vi "newTestStandVariable.vi"(0 "Engine Reference":refnum<k7>, 5 "Sequence File Ref":refnum<k7>, 7 "Variable Type":i32(ring)=1 items=["PropValType_Container", "PropValType_String", "PropValType_Boolean", "PropValType_Number", "PropValType_NamedType", "PropValType_Reference", "PropValType_Array"], 9 "Variable Name":string="Locals.Logs", 11 "error in":errorcluster, 12 "Variable Value":variant, 13 "Array?":bool, 14 "Empty array?":bool) -> (4 "Engine Reference(out)":refnum<k7>, 6 "Sequence File Ref(out)":refnum<k7>, 15 "error out":errorcluster)   [LabVIEW 2010]
doc: "This VI is used to create a TestStand variable. The variable type needs to be specified by selecting the type in the Variable Type enum control."
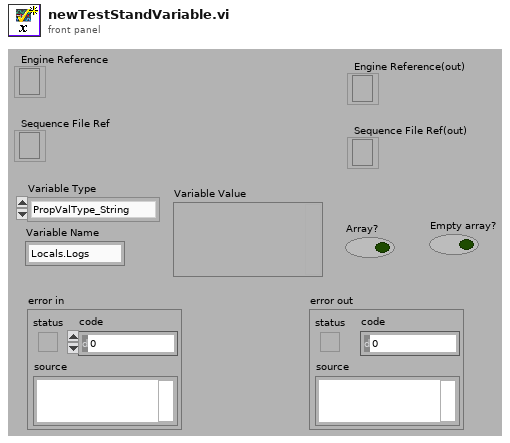
[diagram p1: front panel]
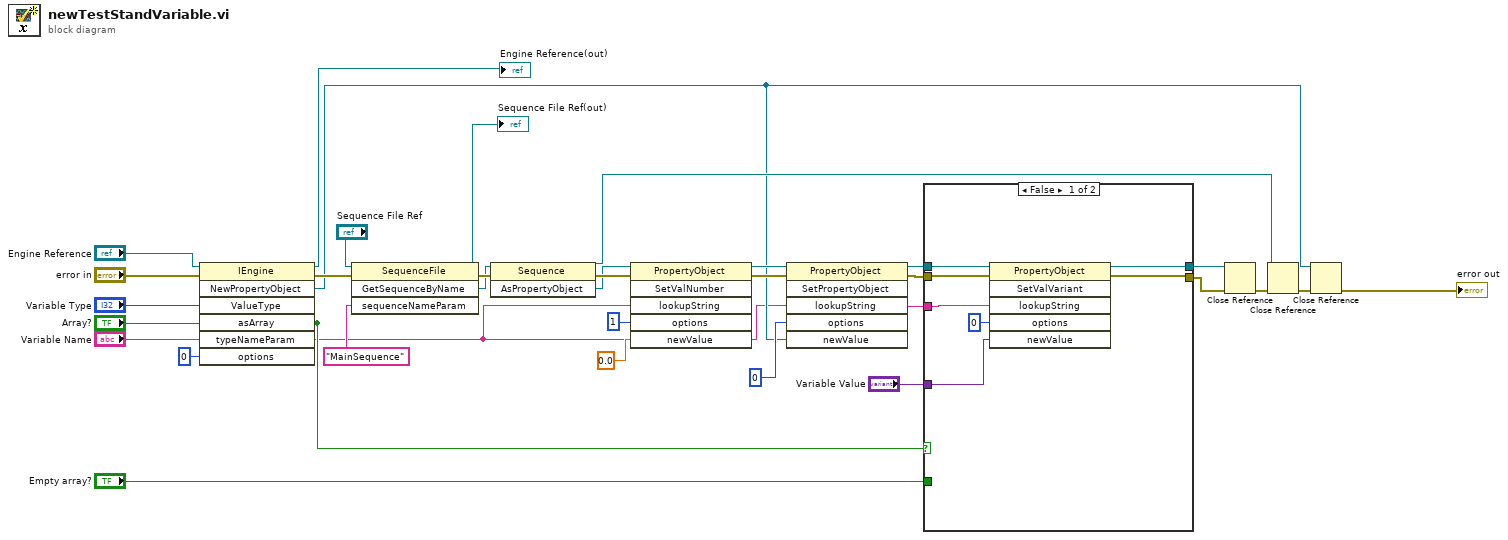
[diagram p0: block diagram]
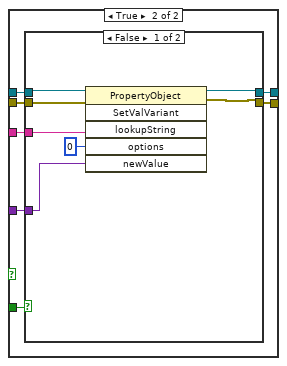
[diagram p2: hidden frame]
diagram:
  n1 = invoke class="IEngine" method="NewPropertyObject"(reference="Engine Reference", error in="error in", "ValueType"="Variable Type", "asArray"="Array?", "typeNameParam"="Variable Name", "options"=0) -> (reference out=→"Engine Reference(out)":refnum<k7>, error out=w11:errorcluster, "NewPropertyObject"=w10:refnum<k7>)  [unwired: 1 in, 4 out]
  n2 = invoke class="SequenceFile" method="GetSequenceByName"(reference="Sequence File Ref", error in=w11, "sequenceNameParam"="MainSequence") -> (reference out=→"Sequence File Ref(out)":refnum<k7>, error out=w17:errorcluster, "GetSequenceByName"=w15:refnum<k7>)  [unwired: 1 in, 1 out]
  n3 = invoke class="Sequence" method="AsPropertyObject"(reference=w15, error in=w17) -> (reference out=w19:refnum<k7>, error out=w13:errorcluster, "AsPropertyObject"=w12:refnum<k7>)  [unwired: 1 in]
  n4 = invoke class="PropertyObject" method="SetValNumber"(reference=w12, error in=w13, "lookupString"="Variable Name", "options"=1, "newValue"=0.0) -> (reference out=w23:refnum<k7>, error out=w21:errorcluster)  [unwired: 1 in, 4 out]
  n5 = invoke class="PropertyObject" method="SetPropertyObject"(reference=w23, error in=w21, "lookupString"="Variable Name", "options"=0, "newValue"=w10) -> (reference out=w8:refnum<k7>, error out=w5:errorcluster)  [unwired: 1 in, 4 out]
  n6 = case shown="False" "Array?" {
    tunnel: w8 -> [w38 w45]
    tunnel: [w37 w44] -> w7
    tunnel: "Empty array?" -> [_ w41]
    tunnel: [w36 w42] -> w4
    tunnel: w5 -> [w35 w43]
    tunnel: "Variable Name" -> [w33 w40]
    tunnel: "Variable Value" -> [w34 w39]
    frame False {
      n7 = invoke class="PropertyObject" method="SetValVariant"(reference=w38, error in=w35, "lookupString"=w33, "options"=0, "newValue"=w34) -> (reference out=w37:refnum<k7>, error out=w36:errorcluster)  [unwired: 1 in, 4 out]
    }
    frame True {
      n8 = case shown="False" w41 {
        tunnel: w45 -> [w52 w54]
        tunnel: [w49 w54] -> w44
        tunnel: w43 -> [w51 w53]
        tunnel: [w48 w53] -> w42
        tunnel: w40 -> [w50 _]
        tunnel: w39 -> [w46 _]
        frame False {
          n9 = invoke class="PropertyObject" method="SetValVariant"(reference=w52, error in=w51, "lookupString"=w50, "options"=0, "newValue"=w46) -> (reference out=w49:refnum<k7>, error out=w48:errorcluster)  [unwired: 1 in, 4 out]
        }
        frame True {
        }
      }
    }
  }
  n10 = Close Reference(reference=w7, error in (no error)=w4) -> (error out=w18:errorcluster)
  n11 = Close Reference(reference=w19, error in (no error)=w18) -> (error out=w24:errorcluster)
  n12 = Close Reference(reference=w10, error in (no error)=w24) -> (error out=→"error out":errorcluster)
